vi "I2C Grove 64x128OLED_SSD1315_Graph.vi"() -> ()   [LabVIEW 2020, in "CTI-Scratchpad.lvlib"]
uses:
  CTI-Scratchpad.lvlib
  CTI/Identity.ctl
  CTI/Error Reporting.ctl
  <vilib>/picture/cartesn2.llb/XY Plot Type.ctl
  CTI/GPIO Number.ctl
  CTI/I2C Number.ctl
  CTI/Session/Session.lvclass
  CTI-Peripheral/I2C OLED/64x128 I2C OLED SSD1315/64x128 I2C OLED SSD1315.lvclass
  CTI/VisaComms/VisaComms.lvclass
  CTI/CTI.lvlib
  <vilib>/ptbypt/NI_PtbyPt.lvlib
panel:
  out "Identity":T1
  in  "stop":bool
  out "2D Picture":picture
  in  "Grove Connector":enum16{"I2C0", "I2C1"}(ring)
  out "error out":errorcluster
  in  "Port":refnum<visa-resource-name>="COM4"
  # "https://wiki.seeedstudio.com/Grove-OLED-Display-0.96-SSD1315/"
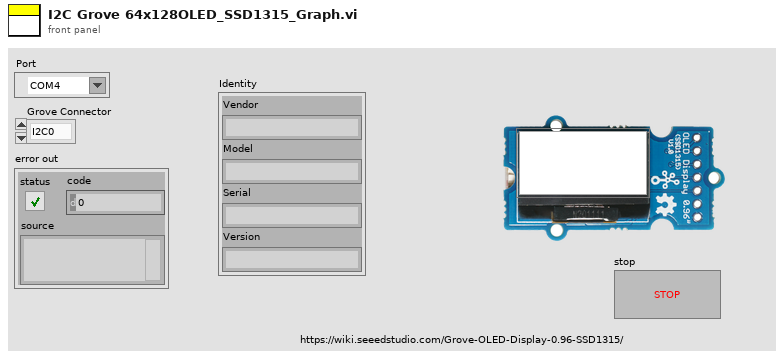
[diagram p1: front panel]
types:
  T1 = typedef "CTI.lvlib/Identity.ctl" = cluster{"Vendor":string, "Model":string, "Serial":string, "Version":string}
  T2 = cluster{"line color":u32, "text color":u32, "tick length(3)":i16, "crossing axes":bool, "visible grid?":bool}
  T3 = cluster{"x minimum":dbl, "x maximum":dbl, "x log?":bool, "x precision":u8, "x format":enum8{"Decimal", "Scientific", "Engineering", "Binary", "Octal", "Hex"}, "y minimum":dbl, "y maximum":dbl, "y log?":bool, "y precision":u8, "y format":enum8{"Decimal", "Scientific", "Engineering", "Binary", "Octal", "Hex"}}
  T4 = typedef "XY Plot Type.ctl" = enum16{"points", "squares", "circles", "connected points", "connected squares", "connected circles", "comb plot", "sized scatter plot", "sized-colored scatter plot", "min-max lines"}
  T5 = cluster{"plot color":u32, "XY plot type":T4, "baseline":dbl}
  T6 = typedef "CTI.lvlib/Error Reporting.ctl" = enum16{"Minimal", "Moderate", "Full"}
  T7 = typedef "CTI.lvlib/I2C Number.ctl" = i8
  T8 = typedef "CTI.lvlib/GPIO Number.ctl" = i8
  T9 = cluster{"horizontal":enum16{"left", "center", "right"}, "vertical":enum16{"top", "center", "bottom"}}
  T10 = cluster{"Font Name:":string, "Size":i16, "Strikeout?":bool, "Italic?":bool, "Underline?":bool, "Outline?":bool, "Shadow?":bool, "Bold?":bool}
  T11 = enum16{"User-specified Font", "Application Font", "System Font", "Dialog Font"}
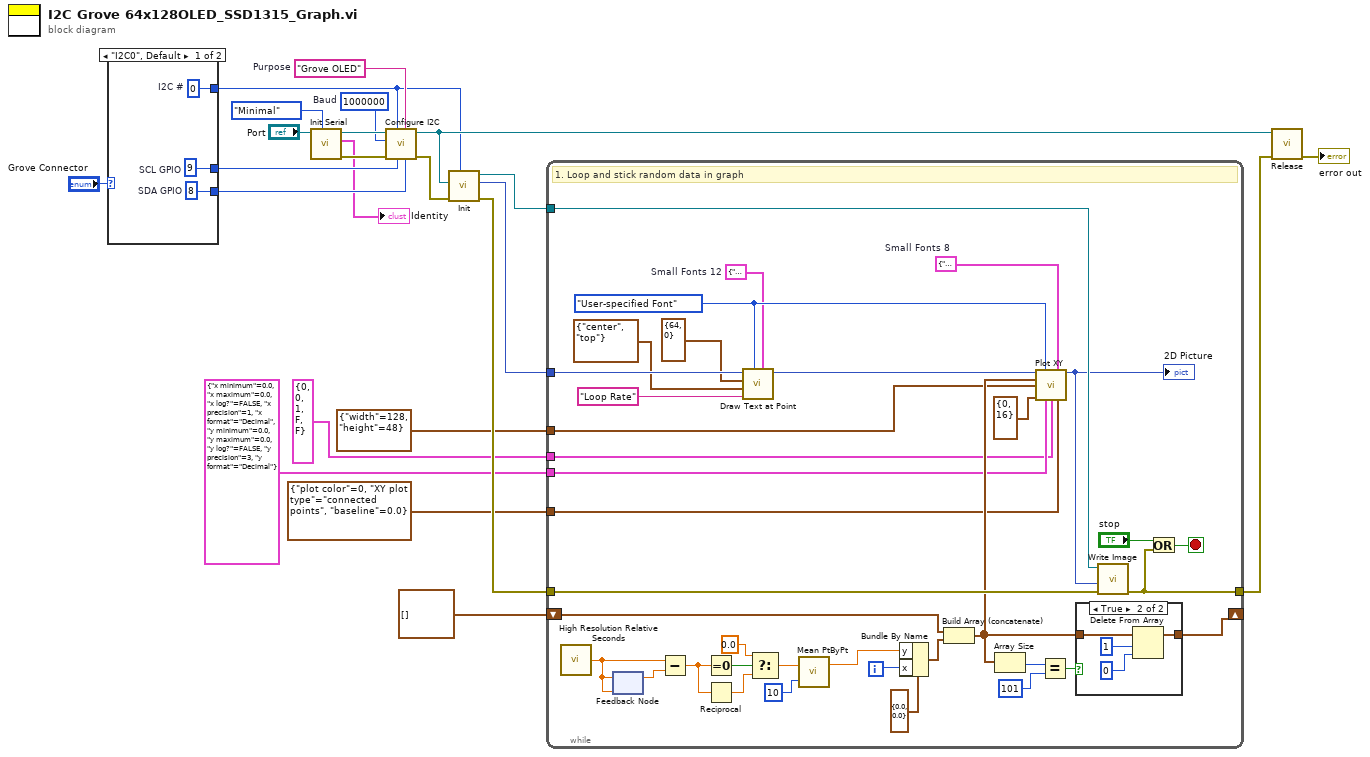
[diagram p0: block diagram]
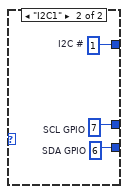
[diagram p3: hidden frame]
diagram:
  w18 = "Grove OLED"  # Purpose
  w19 = u32 1000000  # Baud
  n1 = case shown="\"I2C0\", Default" "Grove Connector" {
    tunnel: [w26 w29] -> w14
    tunnel: [w25 w28] -> w13
    tunnel: [w24 w27] -> w12
    frame "I2C0", Default {
      w24 = T7 0  # I2C #
      w25 = T8 8  # SDA GPIO
      w26 = T8 9  # SCL GPIO
    }
    frame "I2C1" {
      w27 = T7 1  # I2C #
      w28 = T8 6  # SDA GPIO
      w29 = T8 7  # SCL GPIO
    }
  }
  n2 = call "Init Serial.vi"("Error Checking (Full)"=Error_Reporting."Minimal", "VISA resource name in"="Port") -> ("error out"=w20:errorcluster, "Identity"=→"Identity":T1, "Session"=w21:refnum<class "Session.lvclass">)  [unwired: 7 in]
  n3 = call "Configure I2C.vi"("SDA GPIO"=w13, "Purpose (\"I2C\")"=w18, "SCL GPIO"=w14, "I2C #"=w12, "error in (no error)"=w20, "Baud"=w19, "Session in"=w21) -> ("error out"=w17:errorcluster, "Session out"=w16:refnum<class "Session.lvclass">)  [unwired: 3 in]
  n4 = call "Init.vi"("I2C #"=w12, "error in (no error)"=w17, "Session In"=w16) -> ("error out"=w7:errorcluster, "2D Picture"=w9:picture, "64x128 I2C OLED SSD1315 Out"=w8:refnum<class "64x128 I2C OLED SSD1315.lvclass">)  [unwired: 6 in]
  n5 = while {
    tunnel: w9 -> [w66]
    tunnel: w7 -> [w60]
    shift-right: [w52] -> _
    shift-left: cluster{"x":dbl, "y":dbl}[] [] ("data") -> [w63]
    tunnel: w8 -> [w61]
    tunnel: [w37] -> w6
    tunnel: cluster{"width":i16, "height":i16} {"width"=128, "height"=48} ("dimensions (w,h)") -> [w49]
    tunnel: T5 {"plot color"=0, "XY plot type"=enum."connected points", "baseline"=0.0} ("XY plot cosmetics") -> [w48]
    tunnel: T3 {"x minimum"=0.0, "x maximum"=0.0, "x log?"=FALSE, "x precision"=1, "x format"=enum."Decimal", "y minimum"=0.0, "y maximum"=0.0, "y log?"=FALSE, "y precision"=3, "y format"=enum."Decimal"} ("cartesian axis attributes") -> [w47]
    tunnel: T2 {"line color"=0, "text color"=0, "tick length(3)"=1, "crossing axes"=FALSE, "visible grid?"=FALSE} ("cartesian grid cosmetics") -> [w46]
    i -> [w64]
    stop <- w38 stop-if-true
    w39 = T10 {"Font Name:"="Small Fonts", "Size"=12, "Strikeout?"=FALSE, "Italic?"=FALSE, "Underline?"=FALSE, "Outline?"=FALSE, "Shadow?"=FALSE, "Bold?"=FALSE}  # Small Fonts 12
    w40 = T11."User-specified Font" ("desired font(Application)")
    w57 = T10 {"Font Name:"="Small Fonts", "Size"=8, "Strikeout?"=FALSE, "Italic?"=FALSE, "Underline?"=FALSE, "Outline?"=FALSE, "Shadow?"=FALSE, "Bold?"=FALSE}  # Small Fonts 8
    # "1. Loop and stick random data in graph"
    n6 = call <vilib>:"High Resolution Relative Seconds.vi"() -> ("relative seconds"=w51:dbl)
    n7 = feedback-in #1(w51) -> ()
    n8 = feedback #1(w51) -> (w50:dbl)
    n9 = Subtract(x=w51, y=w50) -> (x-y=w32:dbl)
    n10 = Equal To 0?(x=w32) -> (x = 0?=w36:bool)
    n11 = Reciprocal(x=w32) -> (1/x=w35:dbl)
    n12 = call <vilib>:"Draw Text at Point.vi"("[user-specified font]"=w39, "desired font(Application)"=w40, "text"="Loop Rate", "alignment(left, top)"=T9 {"horizontal"=enum."center", "vertical"=enum."top"}, "origin"=cluster{"x":i16, "y":i16} {"x"=64, "y"=0}, "picture"=w66) -> ("new picture"=w44:picture)  [unwired: 4 in, 1 out]
    n13 = Select(t=0.0, s=w36, f=w35) -> (s? t:f=w33:dbl)
    n14 = call <vilib>:"Mean PtByPt.vi"("x"=w33, "sample length"=10) -> ("mean"=w31:dbl)  [unwired: 2 in, 1 out]
    n15 = Bundle By Name(cluster=cluster{"x":dbl, "y":dbl} {"x"=0.0, "y"=0.0} ("Point [horizontal, vertical]"), "y"=w31, "x"=w64) -> (w62:cluster{"x":dbl, "y":dbl})
    n16 = Build Array (concatenate)(w63, w62) -> (w53:cluster{"x":dbl, "y":dbl}[])
    n17 = Array Size(array=w53) -> (size(s)=w56:i32)
    n18 = call <vilib>:"Plot XY.vi"("picture"=w44, "desired font(Application)"=w40, "[user-specified font]"=w57, "data"=w53, "dimensions (w,h)"=w49, "top left point(0, 0)"=cluster{"x":i16, "y":i16} {"x"=0, "y"=16}, "cartesian axis attributes"=w47, "cartesian grid cosmetics"=w46, "XY plot cosmetics"=w48) -> ("new picture"=w58:picture)  [unwired: 6 in]
    "2D Picture" <- w58
    n19 = Equal?(x=w56, y=101) -> (x = y?=w54:bool)
    n20 = case shown="True" w54 {
      tunnel: w53 -> [w67 w71]
      tunnel: [w67 w70] -> w52
      frame False {
      }
      frame True {
        n21 = Delete From Array(array=w71, length=1, index=0) -> (array with subset deleted=w70:cluster{"x":dbl, "y":dbl}[])  [unwired: 1 out]
      }
    }
    n22 = call-dynamic "Write Image.vi"("error in (no error)"=w60, "2D Picture"=w58, "64x128 I2C OLED SSD1315 In"=w61) -> ("error out"=w37:errorcluster)  [unwired: 7 in, 1 out]
    n23 = Or(x="stop", y=w37) -> (x .or. y?=w38:bool)
  }
  n24 = call-dynamic "Release.vi"("error in (no error)"=w6, "Session in"=w16) -> ("error out"=→"error out":errorcluster)  [unwired: 9 in]
